vi "UpdateStatusOnNode.vi"(2 "MyState":T3, 3 "ROS":T1) -> (1 "ROS out":T1)   [LabVIEW 2015]
uses:
  Console/Servers/ServerSubs/MyState.ctl
  _ROSControl.ctl
  _ROSDirection.ctl
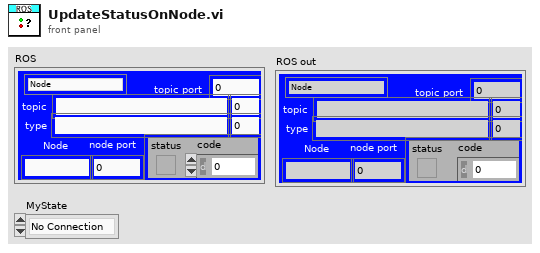
[diagram p1: front panel]
types:
  T1 = typedef "_ROSControl.ctl" = cluster{"topic port":u16, "Node":string, "topic":string, "type":string, "node port":u16, "error ":errorcluster, "Direction":T2, "Update (ms)":u16, "FIFO size":u16}
  T2 = typedef "_ROSDirection.ctl" = enum16{"Node", "Publisher", "Subscriber", "ServiceClient", "ServiceProvider"}
  T3 = typedef "MyState.ctl" = enum16{"No Connection", "Registered", "Connected", "Close"}
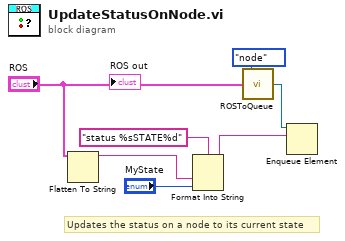
[diagram p0: block diagram]
diagram:
  # "Updates the status on a node to its current state"
  n1 = Flatten To String(anything="ROS") -> (data string=w2:string)  [unwired: 3 in, 2 out]
  n2 = Format Into String(format string="status %sSTATE%d", w2, "MyState") -> (resulting string=w1:string)  [unwired: 2 in, 1 out]
  n3 = call "ROSToQueue.vi"("ROS"="ROS", "Name"=enum16{"topic", "node"}."node") -> ("queue"=w6:refnum<queue>)  [unwired: 2 in, 1 out]
  n4 = Enqueue Element(queue=w6, element=w1) -> ()  [unwired: 2 in, 3 out]
  "ROS out" <- "ROS"
